vi "Button2ToggleV2.1.vi"(1 "a":bool) -> (0 "Result(clone)":bool)   [LabVIEW 2013]
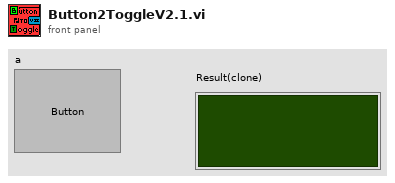
[diagram p1: front panel]
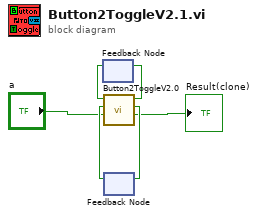
[diagram p0: block diagram]
diagram:
  n1 = feedback #1() -> (w5:bool)  [unwired: 1 in]
  n2 = feedback #2() -> (w3:bool)  [unwired: 1 in]
  n3 = call "Button2ToggleV2.0.vi"("a"="a", "fNodeA(in)"=w3, "fNodeB"=w5) -> ("Result(clone)"=→"Result(clone)":bool, "fNodeA(out)"=w4:bool, "Latched Bool (+fNodeB)"=w6:bool)  [unwired: 6 in]
  n4 = feedback-in #1(w6) -> ()
  n5 = feedback-in #2(w4) -> ()
